vi "Read Event.vi"(8 "error in (no error)":errorcluster caption="entrée d'erreur (pas d'erreur)", 11 "Class Event Shielding Box en entrée":refnum<class "Class Event Balance.lvclass">) -> (0 "error out":errorcluster caption="sortie d'erreur", 3 "Class Event Shielding Box en sortie":refnum<class "Class Event Balance.lvclass">)   [LabVIEW 2020, in "Library Instrument & Equipement.lvlib" / "Library Event.lvlib" / "Class Event Balance.lvclass"]
uses:
  Class Event Balance.lvclass
  C:/Users/ngarcin/OneDrive - Altyor/Standard TB/Class/Core/Actors/Actor_EventStart/Classe Event (Default)/Class Event (Default).lvclass
  JSON API/JSON Value/Set from JSON string.vi
  Instrument/Instrument (Default)/Class Instrument (Default).lvclass
  JSON API/JSON Value/JSON Value.lvclass
  Class Event Balance.lvclass/Class Event Balance.ctl
  JSON API/Variant JSON/Variant JSON.lvlib
  JSON API/Get Polymorphic/JSON GetSet.lvlib
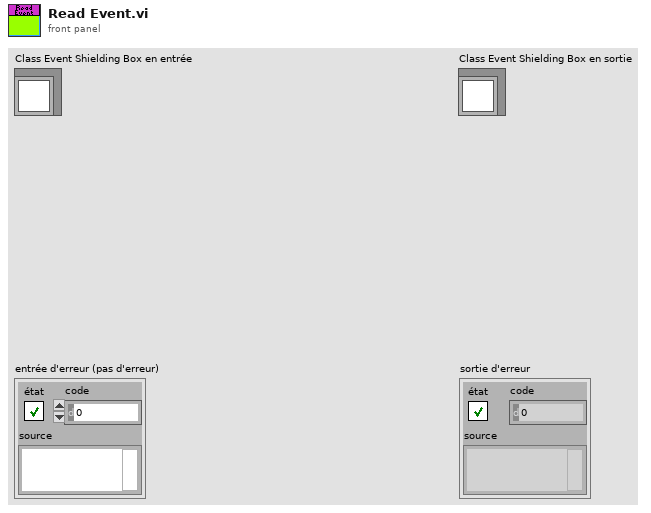
[diagram p1: front panel]
types:
  T1 = cluster{"Weight":dbl, "Front":enum16{"Amount", "Descending"}}
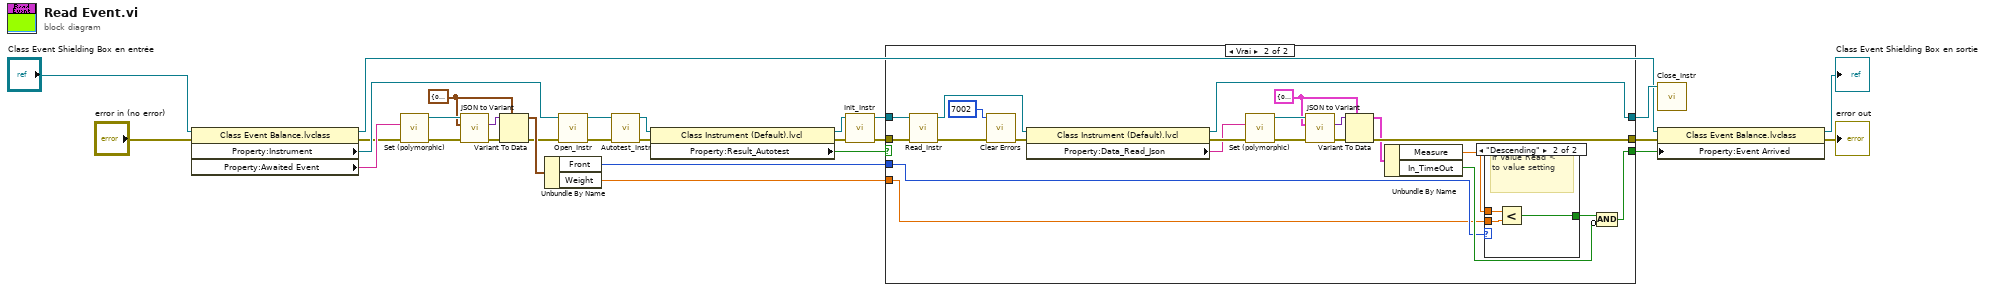
[diagram p0: block diagram]
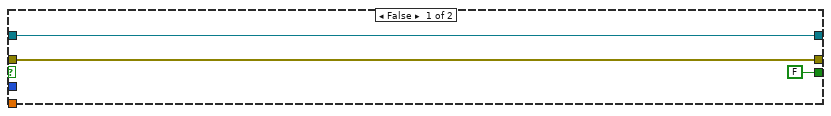
[diagram p2: hidden frame]
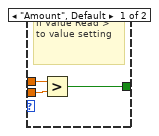
[diagram p3: hidden frame]
diagram:
  w11 = T1 {"Weight"=0.0, "Front"=enum."Descending"}
  n1 = property class="Class Event Balance.lvclass"(reference="Class Event Shielding Box en entrée", error in="error in (no error)") -> (reference out=w21:refnum<class "Class Event Balance.lvclass">, error out=w3:errorcluster, "Property:Instrument"=w6:refnum<class "Class Instrument (Default).lvclass">, "Property:Awaited Event"=w12:string)
  n2 = call-poly "Set (polymorphic).vi"("error in (no error)"=w3, "JSON stream"=w12) -> ("error out"=w15:errorcluster, "JSON Value out"=w17:refnum<class "JSON Value.lvclass">)  [unwired: 7 in, 1 out]
  n3 = call "JSON to Variant.vi"("error in (no error)"=w15, "Variant (Data Type)"=w11, "JSON Value"=w17) -> ("error out"=w16:errorcluster, "Variant out"=w14:variant)  [unwired: 7 in]
  n4 = Variant To Data(error in=w16, type=w11, Variant=w14) -> (data=w13:T1, error out=w2:errorcluster)
  n5 = Unbundle By Name(w13) -> ("Front"=w5:enum16{"Amount", "Descending"}, "Weight"=w4:dbl)
  n6 = call-dynamic "Open_Instr.vi"("error in (no error)"=w2, "Class Multimeter (Default) en entrée"=w6) -> ("error out"=w23:errorcluster, "Class Multimeter (Default) en sortie"=w27:refnum<class "Class Instrument (Default).lvclass">)  [unwired: 8 in]
  n7 = call-dynamic "Autotest_Instr.vi"("error in (no error)"=w23, "Class Instrument (Default) en entrée"=w27) -> ("error out"=w24:errorcluster, "Class Instrument (Default) en sortie"=w26:refnum<class "Class Instrument (Default).lvclass">)  [unwired: 8 in]
  n8 = property class="Class Instrument (Default).lvcl"(reference=w26, error in=w24) -> (reference out=w9:refnum<class "Class Instrument (Default).lvclass">, error out=w8:errorcluster, "Property:Result_Autotest"=w25:bool)
  n9 = call-dynamic "Init_Instr.vi"("error in (no error)"=w8, "Class Instrument (Default) en entrée"=w9) -> ("error out"=w7:errorcluster, "Class Instrument (Default) en sortie"=w10:refnum<class "Class Instrument (Default).lvclass">)  [unwired: 8 in]
  n10 = case shown="Vrai" w25 {
    tunnel: w7 -> [w31 w54]
    tunnel: w10 -> [w32 w53]
    tunnel: [w32 w51] -> w22
    tunnel: [w31 w44] -> w1
    tunnel: [FALSE w37] -> w18
    tunnel: w5 -> [_ w36]
    tunnel: w4 -> [_ w34]
    frame False {
    }
    frame True {
      w40 = cluster{"Measure":dbl, "In_TimeOut":bool} {"Measure"=0.0, "In_TimeOut"=FALSE}
      n11 = call-dynamic "Read_Instr.vi"("error in (no error)"=w54, "Class Instrument (Default) en entrée"=w53) -> ("error out"=w42:errorcluster, "Class Instrument (Default) en sortie"=w52:refnum<class "Class Instrument (Default).lvclass">)  [unwired: 8 in]
      n12 = call <vilib>:"Clear Errors.vi"("error in (no error)"=w42, "specific error code to clear (0: all)"=7002) -> ("error out"=w41:errorcluster)  [unwired: 4 in, 1 out]
      n13 = property class="Class Instrument (Default).lvcl"(reference=w52, error in=w41) -> (reference out=w51:refnum<class "Class Instrument (Default).lvclass">, error out=w46:errorcluster, "Property:Data_Read_Json"=w45:string)
      n14 = call-poly "Set (polymorphic).vi"("error in (no error)"=w46, "JSON stream"=w45) -> ("error out"=w49:errorcluster, "JSON Value out"=w47:refnum<class "JSON Value.lvclass">)  [unwired: 7 in, 1 out]
      n15 = call "JSON to Variant.vi"("error in (no error)"=w49, "Variant (Data Type)"=w40, "JSON Value"=w47) -> ("error out"=w48:errorcluster, "Variant out"=w50:variant)  [unwired: 7 in]
      n16 = Variant To Data(error in=w48, type=w40, Variant=w50) -> (data=w39:cluster{"Measure":dbl, "In_TimeOut":bool}, error out=w44:errorcluster)
      n17 = Unbundle By Name(w39) -> ("Measure"=w35:dbl, "In_TimeOut"=w38:bool)
      n18 = case shown="\"Descending\"" w36 {
        tunnel: w35 -> [w57 w60]
        tunnel: w34 -> [w56 w59]
        tunnel: [w55 w58] -> w33
        frame "Amount", Default {
          # "If Value Read > to value setting"
          n19 = Greater?(x=w57, y=w56) -> (0:w55:bool)
        }
        frame "Descending" {
          # "If Value Read < to value setting"
          n20 = Less?(x=w60, y=w59) -> (x < y?=w58:bool)
        }
      }
      n21 = Compound Arithmetic op=AND(w33, invert w38) -> (w37:bool)
    }
  }
  n22 = call-dynamic "Close_Instr.vi"("Class Instrument (Default) en entrée"=w22) -> ()  [unwired: 9 in, 2 out]
  n23 = property class="Class Event Balance.lvclass"(reference=w21, error in=w1, "Property:Event Arrived"=w18) -> (reference out=→"Class Event Shielding Box en sortie":refnum<class "Class Event Balance.lvclass">, error out=→"error out":errorcluster)
